vi "Centrialize Error Handler.vi"(8 "error in (no error)":errorcluster, 9 "Error":errorcluster, 10 "Error Level":T1, 11 "ATM Controller in":refnum<class "ATM Controller.lvclass">) -> (0 "error out":errorcluster, 3 "ATM Controller out":refnum<class "ATM Controller.lvclass">)   [LabVIEW 2019, in "ATM Controller.lvlib" / "ATM Controller.lvclass"]
uses:
  ATM Controller.lvclass
  <vilib>/ActorFramework/Actor/Actor.lvclass
  ATM Controller Messages/Set State Msg/Set State Msg.lvclass
  State -Enum.ctl
  C:/Program Files (x86)/National Instruments/LabVIEW 2019/vi.lib/ActorFramework/Actor/Actor.lvclass
  Error Level.ctl
  Error Data.ctl
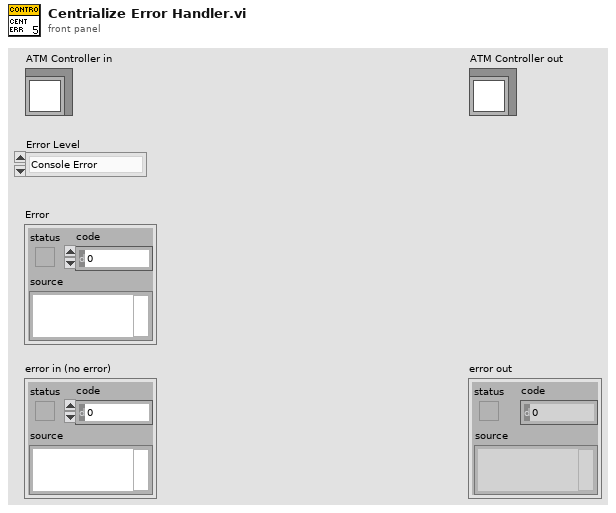
[diagram p1: front panel]
types:
  T1 = typedef "ATM Controller.lvlib/ATM Controller.lvclass/Error Level.ctl" = enum16{"Console Error", "Sensor Interface Error", "Process Step Error"}
  T2 = typedef "ATM Controller.lvlib/ATM Controller.lvclass/Error Data.ctl" = cluster{"Description":string, "Error Level":T1, "Time Stamp":timestamp}
  T3 = typedef "ATM Controller.lvlib/ATM Controller.lvclass/State -Enum.ctl" = enum16{"Inital", "Idle", "Login", "Balance Inquiry", "Deposit", "Withdrawal", "Fast Cash", "Terminate"}
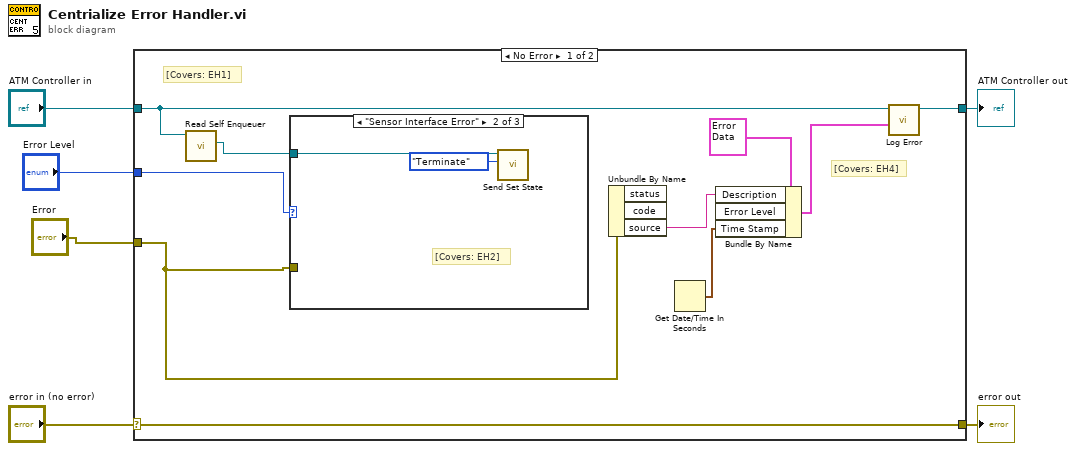
[diagram p0: block diagram]
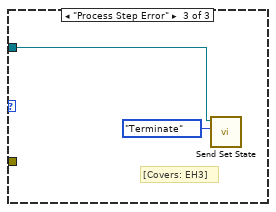
[diagram p3: hidden frame]
diagram:
  n1 = case shown="No Error" "error in (no error)" {
    selector: "error in (no error)" -> [w16 w22]
    tunnel: [w16 w22] -> w5
    tunnel: [w12 w21] -> w3
    tunnel: "ATM Controller in" -> [w13 w21]
    tunnel: "Error" -> [w7 _]
    tunnel: "Error Level" -> [w15 _]
    frame No Error {
      # "[Covers: EH4]"
      # "[Covers: EH1]"
      n2 = call <vilib>:"Read Self Enqueuer.vi"("Actor"=w13) -> ("Self Enqueuer"=w14:refnum<class "Message Enqueuer.lvclass">)  [unwired: 10 in]
      n3 = case shown="\"Sensor Interface Error\"" w15 {
        tunnel: w14 -> [_ w18 w19]
        tunnel: w7 -> [_ _ _]
        frame "Console Error", Default {
        }
        frame "Sensor Interface Error" {
          # "[Covers: EH2]"
          n4 = call "Send Set State.vi"("State"=State_-Enum."Terminate", "Message Enqueuer"=w18) -> ()  [unwired: 8 in, 2 out]
        }
        frame "Process Step Error" {
          # "[Covers: EH3]"
          n5 = call "Send Set State.vi"("State"=State_-Enum."Terminate", "Message Enqueuer"=w19) -> ()  [unwired: 8 in, 2 out]
        }
      }
      n6 = Unbundle By Name(w7) -> ("source"=w9:string)  [unwired: 2 out]
      n7 = Get Date/Time In Seconds() -> (seconds since 1Jan1904=w10:timestamp)
      n8 = Bundle By Name(cluster=T2 {"Description"="", "Error Level"=enum."Console Error", "Time Stamp"=timestamp(0 s since 1904-01-01)} ("Error Data"), "Description"=w9, "Time Stamp"=w10) -> (w8:T2)  [unwired: 1 in]
      n9 = call "Log Error.vi"("Error Data"=w8, "ATM Controller in"=w13) -> ("ATM Controller out"=w12:refnum<class "ATM Controller.lvclass">)  [unwired: 8 in, 1 out]
    }
    frame Error {
    }
  }
  "error out" <- w5
  "ATM Controller out" <- w3
